vi "Test_Calculate Pull-in.vi"(6 "Amps":T2 format="%5.3f A", 9 "Volts":T1 format="%5.3f V", 10 "V_MAX":dbl, 11 "Table in":refnum<vi>) -> ()   [LabVIEW 2025]
uses:
  Controls/Numeric Current.ctl
  Controls/Numeric Voltage.ctl
panel:
  out "concatenated string":string
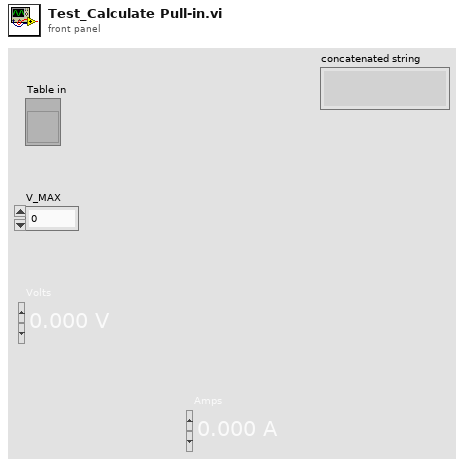
[diagram p1: front panel]
types:
  T1 = typedef "Numeric Voltage.ctl" = dbl
  T2 = typedef "Numeric Current.ctl" = dbl
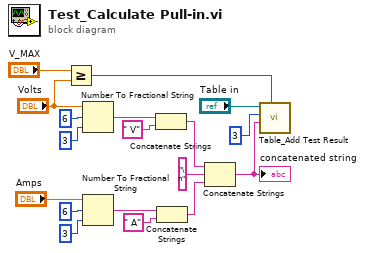
[diagram p0: block diagram]
diagram:
  n1 = Greater Or Equal?(x="V_MAX", y="Volts") -> (x >= y?=w2:bool)
  n2 = Number To Fractional String(number="Volts", width (-)=i16 6, precision (6)=i16 3) -> (F-format string=w14:string)  [unwired: 1 in]
  n3 = Number To Fractional String(number="Amps", width (-)=i16 6, precision (6)=i16 3) -> (F-format string=w11:string)  [unwired: 1 in]
  n4 = Concatenate Strings(w14, " V" ("string")) -> (w10:string)
  n5 = Concatenate Strings(w11, " A" ("string")) -> (w9:string)
  n6 = Concatenate Strings(w10, "\n" ("string"), w9) -> (w3:string)
  "concatenated string" <- w3
  n7 = call "Table_Add Test Result.vi"("Pass?"=w2, "Test Result"=w3, "index (row)"=3, "Table in"="Table in") -> ()  [unwired: 7 in, 1 out]
